vi "Write size.vi"(8 "error in (no error)":errorcluster, 10 "size":u64, 11 "file attributes in":refnum<class "File Attributes.lvclass">) -> (0 "error out":errorcluster, 3 "file attributes out":refnum<class "File Attributes.lvclass">)   [LabVIEW 2020, in "NI_SFTP.lvlib" / "File Attributes.lvclass"]
doc: "Writes a file size (in bytes) to this File Attributes object. Use this property with <b>Set File Attributes</b> to set the file size of a remote file."
uses:
  <vilib>/net/SFTP/File Attributes/File Attributes.lvclass
  <vilib>/net/SFTP/File Attributes/File Attributes.lvclass/File Attributes.ctl
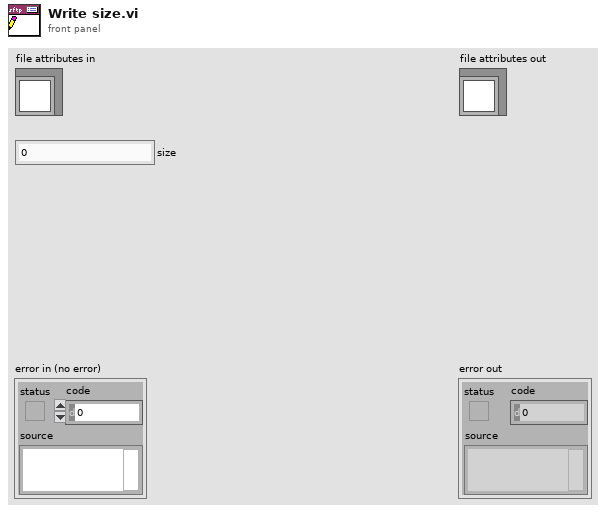
[diagram p1: front panel]
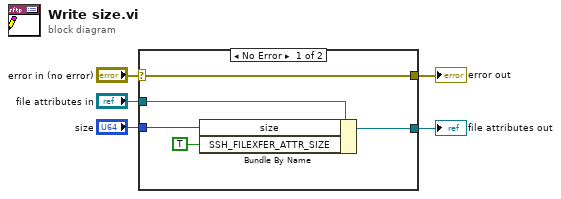
[diagram p0: block diagram]
diagram:
  n1 = case shown="No Error" "error in (no error)" {
    selector: "error in (no error)" -> [w10 w11]
    tunnel: [w10 w11] -> w4
    tunnel: [w8 w12] -> w2
    tunnel: "file attributes in" -> [w9 w12]
    tunnel: "size" -> [w7 _]
    frame No Error {
      n2 = Bundle By Name(cluster=w9, "size"=w7, "SSH_FILEXFER_ATTR_SIZE"=TRUE ("SFTP Session.lvclass:Name.File Attributes.SSH_FILEXFER_ATTR_SIZE")) -> (w8:refnum<class "File Attributes.lvclass">)
    }
    frame Error {
    }
  }
  "error out" <- w4
  "file attributes out" <- w2
